vi "Button and stepper (SILAR).vi"(0 "Arduino Resource In":T1={"VISA resource"="", "Board Type"=enum."Uno", "Connection Type"=enum."USB / Serial", "Bytes Per Packet (15)"=15}, 1 "Шаговый двигатель №":u8, 5 "Кол-во шагов":i16, 9 "Скорость двигателя":i16=100, 11 "Error In":errorcluster, 12 "Контакт концевика":u8, 14 "ENABLE контакт":u8) -> (4 "Arduino Resource Out":T1={"VISA resource"="", "Board Type"=enum."Uno", "Connection Type"=enum."USB / Serial", "Bytes Per Packet (15)"=15}, 15 "Error Out":errorcluster)   [LabVIEW 2016]
uses:
  <vilib>/LabVIEW Interface for Arduino/Type Defs/Arduino Resource.ctl
  <vilib>/LabVIEW Interface for Arduino/Type Defs/Board Type.ctl
  <vilib>/LabVIEW Interface for Arduino/LabVIEW Interface for Arduino.lvlib
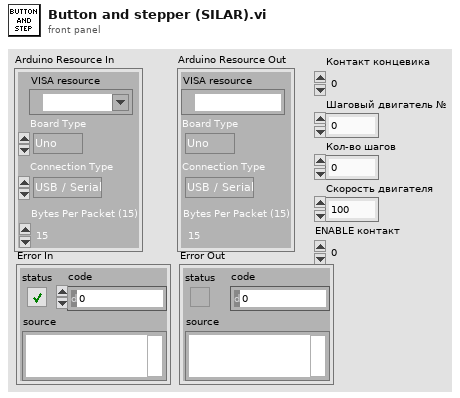
[diagram p1: front panel]
types:
  T1 = typedef "LabVIEW Interface for Arduino.lvlib/Arduino Resource.ctl" = cluster{"VISA resource":refnum<visa-resource-name>, "Board Type":T2, "Connection Type":enum8{"USB / Serial"}, "Bytes Per Packet (15)":u8}
  T2 = typedef "LabVIEW Interface for Arduino.lvlib/Board Type.ctl" = enum16{"Uno", "Dimuelanove w/Atmega 328", "Mega 2560"}
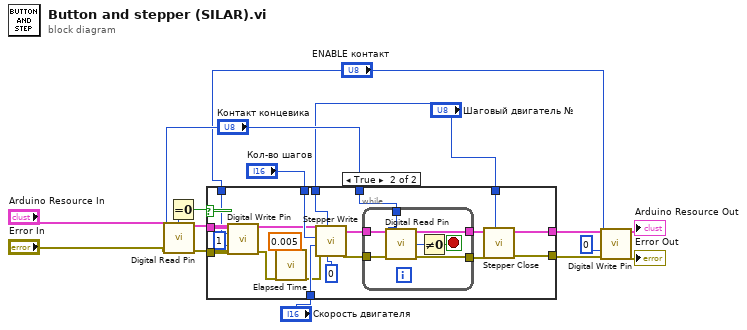
[diagram p0: block diagram]
diagram:
  n1 = call <vilib>:"Digital Read Pin.vi"("Arduino Resource"="Arduino Resource In", "Digital I/O Pin (0)"="Контакт концевика", "error in"="Error In") -> ("Arduino Resource"=w14:T1, "Value"=w9:u8, "error out"=w13:errorcluster)  [unwired: 10 in]
  n2 = Equal To 0?(x=w9) -> (x = 0?=w10:bool)
  n3 = case shown="True" w10 {
    tunnel: "Скорость двигателя" -> [_ w34]
    tunnel: "Кол-во шагов" -> [_ w33]
    tunnel: "Шаговый двигатель №" -> [_ w32]
    tunnel: w14 -> [w18 w23]
    tunnel: w13 -> [w17 w22]
    tunnel: "Контакт концевика" -> [_ w38]
    tunnel: [w18 w29] -> w5
    tunnel: [w17 w28] -> w4
    tunnel: "Шаговый двигатель №" -> [_ w27]
    tunnel: "ENABLE контакт" -> [_ w21]
    frame False {
    }
    frame True {
      n4 = call <vilib>:"Digital Write Pin.vi"("Arduino Resource"=w23, "Digital I/O Pin (0)"=w21, "Value (0)"=u8 1, "error in"=w22) -> ("Arduino Resource"=w20:T1, "error out"=w25:errorcluster)  [unwired: 10 in]
      n5 = call "Elapsed Time"("Time Target (s)"=0.005, "error in (no error)"=w25) -> ("error out"=w19:errorcluster)  [unwired: 10 in, 7 out]
      n6 = call <vilib>:"Stepper Write.vi"("Set Acceleration (0 to disable)"=i16 0, "Stepper #"=w32, "error in"=w19, "Set Speed (Steps per Second)"=w34, "# of Steps to Move"=w33, "Arduino Resource"=w20) -> ("error out"=w36:errorcluster, "Arduino Resource Out"=w37:T1)  [unwired: 4 in]
      n7 = while {
        tunnel: [w45] -> w30
        tunnel: [w44] -> w31
        tunnel: w38 -> [w43]
        tunnel: w37 -> [w40]
        tunnel: w36 -> [w39]
        stop <- w41 stop-if-true
        n8 = call <vilib>:"Digital Read Pin.vi"("Arduino Resource"=w40, "Digital I/O Pin (0)"=w43, "error in"=w39) -> ("Arduino Resource"=w45:T1, "Value"=w42:u8, "error out"=w44:errorcluster)  [unwired: 10 in]
        n9 = Not Equal To 0?(x=w42) -> (x != 0?=w41:bool)
      }
      n10 = call <vilib>:"Stepper Close.vi"("Stepper #"=w27, "error in"=w31, "Arduino Resource"=w30) -> ("error out"=w28:errorcluster, "Arduino Resource Out"=w29:T1)  [unwired: 7 in]
    }
  }
  n11 = call <vilib>:"Digital Write Pin.vi"("Arduino Resource"=w5, "Digital I/O Pin (0)"="ENABLE контакт", "Value (0)"=u8 0, "error in"=w4) -> ("Arduino Resource"=→"Arduino Resource Out":T1, "error out"=→"Error Out":errorcluster)  [unwired: 10 in]
